vi "Import Spreadsheet.vi"(6 "delimiter (\\t)":string="\t", 7 "format (%.3f)":string="%.3f", 8 "error in (no error)":errorcluster, 11 "file path (dialog if empty)":path) -> (0 "error out":errorcluster, 3 "Problem out":T1)   [LabVIEW 2015]
doc: "Imports a delimited file to an svm_problem.\nFirst column is assumed to be the label, while the remaining columns are the features."
uses:
  LibSVM Sparse/Wrapper API/Controls/svm_problem.ctl
  LibSVM Sparse/Wrapper API/Controls/svm_node.ctl
  <userlib>/_OpenG.lib/file/file.llb/Valid Path - Traditional__ogtk.vi
  <vilib>/Utility/file.llb/Read From Spreadsheet File (DBL).vi
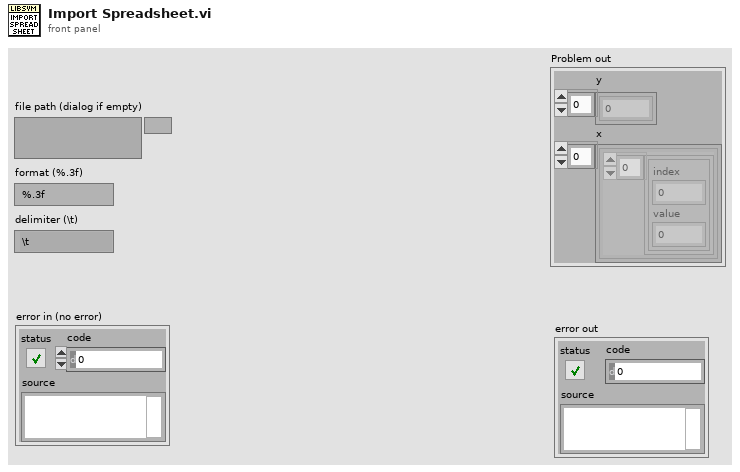
[diagram p1: front panel]
types:
  T1 = typedef "svm_problem.ctl" = cluster{"y":dbl[], "x":cluster{T2[]}[]}
  T2 = typedef "svm_node.ctl" = cluster{"index":i32, "value":dbl}
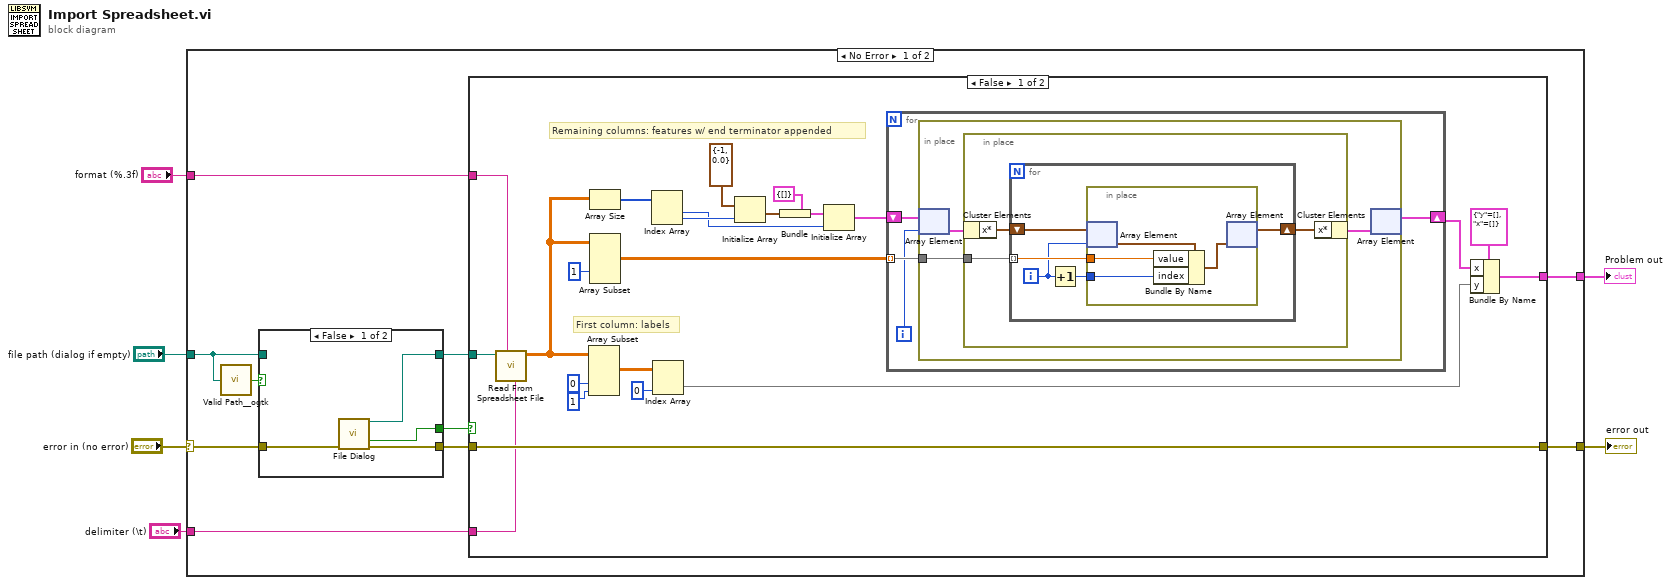
[diagram p0: block diagram]
diagram:
  n1 = case shown="No Error" "error in (no error)" {
    selector: "error in (no error)" -> [w15 w66]
    tunnel: "delimiter (\\t)" -> [w7 _]
    tunnel: [w10 w66] -> w5
    tunnel: "file path (dialog if empty)" -> [w14 _]
    tunnel: [w12 _] -> w2
    tunnel: "format (%.3f)" -> [w8 _]
    frame No Error {
      n2 = call-poly <userlib>:"Valid Path__ogtk.vi"("path"=w14) -> ("valid"=w16:bool)
      n3 = case shown="False" w16 {
        tunnel: w15 -> [w63 w64]
        tunnel: [w62 w64] -> w11
        tunnel: w14 -> [_ w65]
        tunnel: [w61 w65] -> w13
        tunnel: [w60 _] -> w9
        frame False {
          n4 = call "File Dialog"("error in"=w63) -> ("selected path"=w61:path, "cancelled"=w60:bool, "error out"=w62:errorcluster)  [unwired: 11 in, 1 out]
        }
        frame True {
        }
      }
      n5 = case shown="False" w9 {
        tunnel: w13 -> [w21 _]
        tunnel: [w20 _] -> w12
        tunnel: w11 -> [w19 w59]
        tunnel: [w19 w59] -> w10
        tunnel: w8 -> [w18 _]
        tunnel: w7 -> [w17 _]
        frame False {
          # "Remaining columns: features w/ end terminator appended"
          # "First column: labels"
          n6 = call-poly <vilib>:"Read From Spreadsheet File.vi"("delimiter (\\t)"=w17, "format (%.3f)"=w18, "file path (dialog if empty)"=w21) -> ("all rows"=w31:dbl[][])  [unwired: 4 in, 4 out]
          n7 = Array Subset(array=w31, index (col)=0 ("index"), length (col)=1 ("length")) -> (w34:dbl[][])  [unwired: 2 in]
          n8 = Array Size(array=w31) -> (size(s)=w30:i32[])
          n9 = Array Subset(array=w31, index (col)=1 ("index")) -> (w23:dbl[][])  [unwired: 3 in]
          n10 = Index Array(array=w30) -> (element #1=w26:i32, element #2=w29:i32)  [unwired: 2 in]
          n11 = Index Array(array=w34, index (col)=0 ("disabled index (col)")) -> (element=w32:dbl[])  [unwired: 1 in]
          n12 = Initialize Array(T2 {"index"=-1, "value"=0.0} ("svm_node"), w29) -> (w28:T2[])
          n13 = Bundle(cluster=cluster{"x*":T2[]} {"x*"=[]}, "x*"=w28) -> (w27:cluster{"x*":T2[]})
          n14 = Initialize Array(w27, w26) -> (w25:cluster{"x*":T2[]}[])
          n15 = for {
            tunnel: w23 -> [w43] mode=indexing
            shift-right: [w40] -> w35
            shift-left: w25 -> [w42]
            i -> [w41]
            n16 = in-place {
              in-place-border: w43 -> [w46]
              n17 = in-place-array #1(w42, w41) -> (w45:cluster{"x*":T2[]})
              n18 = in-place {
                in-place-border: w46 -> [w49]
                n19 = in-place-cluster #2(w45) -> ("x*"=w48:T2[])
                n20 = for {
                  tunnel: w49 -> [w54] mode=indexing
                  shift-right: [w50] -> w47
                  shift-left: w48 -> [w51]
                  i -> [w52]
                  n21 = Increment(x=w52) -> (x+1=w53:i32)
                  n22 = in-place {
                    in-place-border: w54 -> [w58]
                    in-place-border: w53 -> [w57]
                    n23 = in-place-array #3(w51, w52) -> (w56:T2)
                    n24 = Bundle By Name(cluster=w56, "value"=w58, "index"=w57) -> (w55:T2)
                    n25 = in-place-array #3(w55) -> (w50:T2[])  [unwired: 1 out]
                  }
                }
                n26 = in-place-cluster #2("x*"=w47) -> (w44:cluster{"x*":T2[]})
              }
              n27 = in-place-array #1(w44) -> (w40:cluster{"x*":T2[]}[])  [unwired: 1 out]
            }
          }
          n28 = Bundle By Name(cluster=T1 {"y"=[], "x"=[]} ("Problem"), "x"=w35, "y"=w32) -> (w20:T1)
        }
        frame True {
          # "Cancelled file dialog"
        }
      }
    }
    frame Error {
    }
  }
  "Problem out" <- w2
  "error out" <- w5
